vi "TCP.IP Server for Ripple Detection - Experiment 3.vi"() -> ()   [LabVIEW 2021]
doc: "Demonstrates how to set up a basic TCP connection, send data to the specified port once a connection has been established, and terminate the connection once the data has been sent. This VI is designed to stop if the TCP connection is terminated. The data sent in this example is an array of random numbers."
panel:
  in  "Number of row to read \nat a time":i32=10000
  in  "File Path":path
  out "Iteration terminal":i32
  in  "Stop 2":bool
  in  "Client Closed":string="The client VI closed the connection."
  in  "Stop":bool
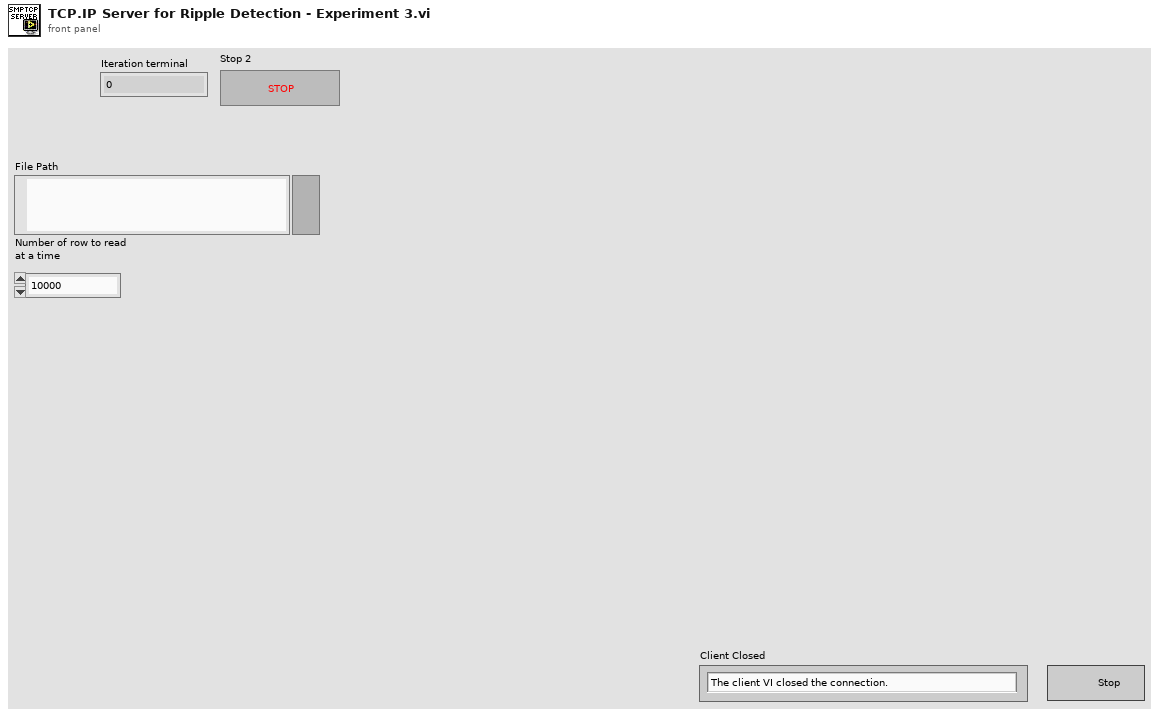
[diagram p1: front panel]
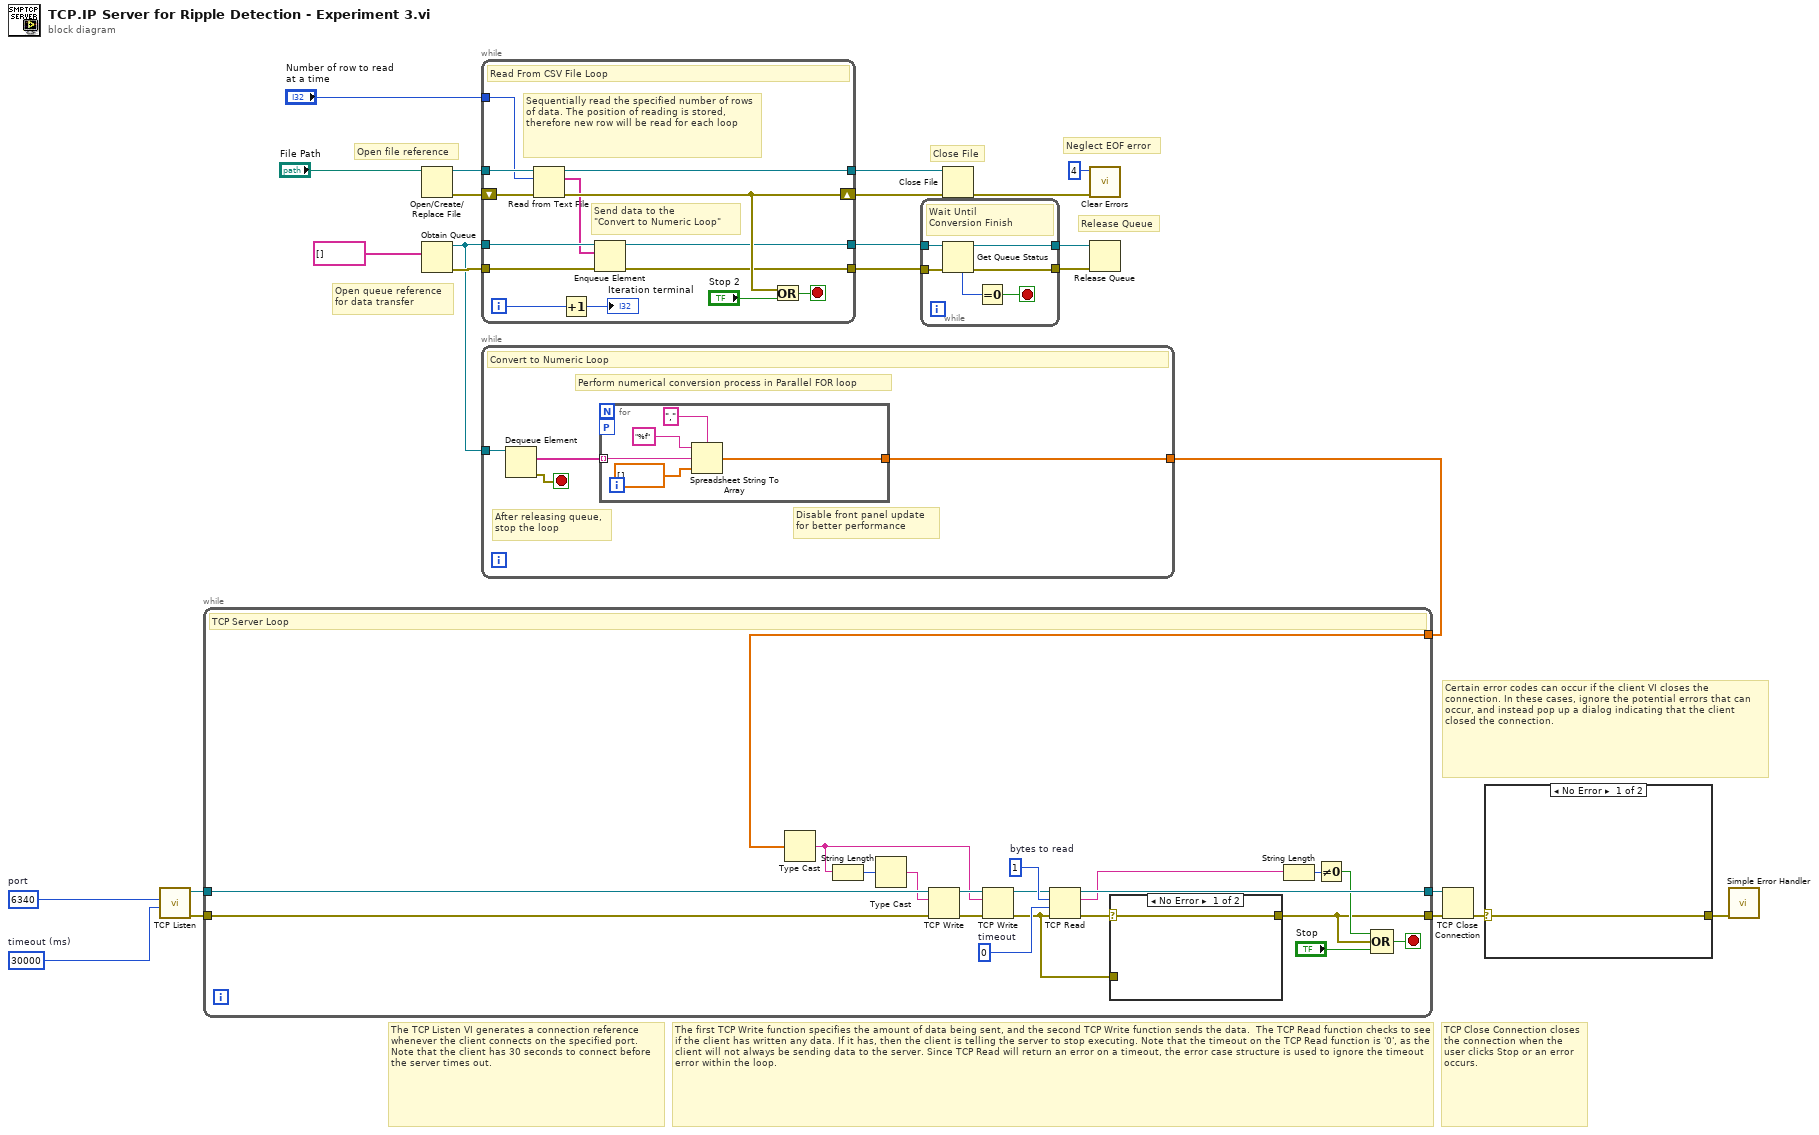
[diagram p0: block diagram]
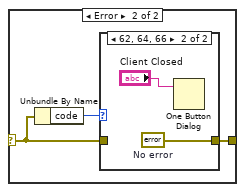
[diagram p2: hidden frame]
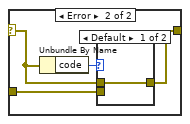
[diagram p4: hidden frame]
diagram:
  w17 = u16 6340  # port
  w18 = 30000  # timeout (ms)
  # "Neglect EOF error"
  # "Release Queue"
  # "Close File"
  # "Open queue reference\nfor data transfer"
  # "Open file reference"
  # "TCP Close Connection closes the connection when the user clicks Stop or an error occurs."
  # "The TCP Listen VI generates a connection reference whenever the client connects on the specified port. Note that the client has 30 seconds to connect before the server times out."
  # "Certain error codes can occur if the client VI closes the connection. In these cases, ignore the potential errors that can occur, and instead pop up a dialog indicating that the client closed the connection."
  # "The first TCP Write function specifies the amount of data being sent, and the second TCP Write function sends the data.  The TCP Read function checks to see if the client has written any data. If it has, then the client is telling the server to stop executing. Note that the timeout on the TCP Read function is '0', as the client will not always be sending data to the server. Since TCP Read will return an error on a timeout, the error case structure is used to ignore the timeout error within the loop."
  n1 = call <vilib>:"TCP Listen.vi"("timeout ms (wait forever: -1)"=w18, "port"=w17) -> ("error out"=w19:errorcluster, "connection ID"=w20:refnum<k5>)  [unwired: 5 in, 3 out]
  n2 = Open/Create/Replace File(file path (use dialog)="File Path") -> (refnum out=w14:refnum<file>, error out=w13:errorcluster)  [unwired: 5 in, 1 out]
  n3 = Obtain Queue(element data type=string[] [] ("形式文字列")) -> (queue out=w6:refnum<queue>, error out=w7:errorcluster)  [unwired: 4 in, 1 out]
  n4 = while {
    tunnel: w14 -> [w38]
    tunnel: [w36] -> w11
    shift-right: [w31] -> w10
    shift-left: w13 -> [w37]
    tunnel: "Number of row to read \nat a time" -> [w32]
    tunnel: w6 -> [w30]
    tunnel: w7 -> [w29]
    tunnel: [w27] -> w5
    tunnel: [w26] -> w4
    i -> [w34]
    stop <- w35 stop-if-true
    # "Send data to the \n\"Convert to Numeric Loop\""
    # "Sequentially read the specified number of rows of data. The position of reading is stored, therefore new row will be read for each loop"
    # "Read From CSV File Loop"
    n5 = Read from Text File(file (use dialog)=w38, count=w32, error in=w37) -> (refnum out=w36:refnum<file>, text=w28:string[], error out=w31:errorcluster)  [unwired: 1 in, 1 out]
    n6 = Increment(x=w34) -> (x+1=→"Iteration terminal":i32)
    n7 = Enqueue Element(queue=w30, element=w28, error in (no error)=w29) -> (queue out=w27:refnum<queue>, error out=w26:errorcluster)  [unwired: 1 in, 1 out]
    n8 = Or(x=w31, y="Stop 2") -> (x .or. y?=w35:bool)
  }
  n9 = while {
    tunnel: w6 -> [w42]
    tunnel: [w39] -> w1
    stop <- w40 stop-if-true
    # "Disable front panel update \nfor better performance"
    # "After releasing queue,\nstop the loop"
    # "Perform numerical conversion process in Parallel FOR loop"
    # "Convert to Numeric Loop"
    n10 = Dequeue Element(queue=w42) -> (element=w41:string[], error out=w40:errorcluster)  [unwired: 2 in, 2 out]
    n11 = for "Forループ" {
      tunnel: w41 -> [w45] mode=indexing
      tunnel: [w43] -> w39
      workers-P: _ -> [_]
      n12 = Spreadsheet String To Array(delimiter (Tab)="," ("デリミタ（タブ）"), format string="%f" ("形式文字列"), spreadsheet string=w45, array type (2D Dbl)=dbl[] []) -> (array=w43:dbl[])
    }
  }
  n13 = while {
    tunnel: [w50] -> w23
    tunnel: [w56] -> w24
    tunnel: w20 -> [w67]
    tunnel: w19 -> [w60]
    tunnel: w1 -> [w48]
    stop <- w61 stop-if-true
    w55 = 0  # timeout
    w58 = 1  # bytes to read
    # "TCP Server Loop"
    n14 = Type Cast(x=w48) -> (*(type *) &x=w62:string)  [unwired: 1 out]
    n15 = String Length(string=w62) -> (length=w64:i32)
    n16 = Type Cast(x=w64) -> (*(type *) &x=w63:string)  [unwired: 1 out]
    n17 = TCP Write(connection ID=w67, data in=w63, error in (no error)=w60) -> (connection ID out=w66:refnum<k5>, error out=w65:errorcluster)  [unwired: 2 out]
    n18 = TCP Write(connection ID=w66, data in=w62, error in (no error)=w65) -> (connection ID out=w57:refnum<k5>, error out=w49:errorcluster)  [unwired: 2 out]
    n19 = TCP Read(connection ID=w57, bytes to read=w58, error in (no error)=w49, 9:w55) -> (connection ID out=w56:refnum<k5>, data out=w53:string, error out=w51:errorcluster)  [unwired: 1 out]
    n20 = case shown="No Error" w51 {
      selector: w51 -> [w68 w71]
      tunnel: [w68 w69] -> w50
      tunnel: w49 -> [_ w70]
      frame No Error {
      }
      frame Error {
        n21 = Unbundle By Name(w71) -> ("code"=w72:i32)
        n22 = case shown="Default" w72 {
          tunnel: w71 -> [w73 _]
          tunnel: w70 -> [_ w74]
          tunnel: [w73 w74] -> w69
          frame Default {
          }
          frame 56 {
          }
        }
      }
    }
    n23 = String Length(string=w53) -> (length=w54:i32)
    n24 = Not Equal To 0?(x=w54) -> (x != 0?=w52:bool)
    n25 = Compound Arithmetic op=OR(w52, w50, "Stop") -> (w61:bool)
  }
  n26 = while {
    tunnel: w5 -> [w80]
    tunnel: w4 -> [w79]
    tunnel: [w76] -> w2
    tunnel: [w75] -> w3
    stop <- w77 stop-if-true
    # "Wait Until \nConversion Finish"
    n27 = Get Queue Status(queue=w80, error in (no error)=w79) -> (queue out=w76:refnum<queue>, error out=w75:errorcluster, # elements in queue=w78:i32)  [unwired: 1 in, 5 out]
    n28 = Equal To 0?(x=w78) -> (x = 0?=w77:bool)
  }
  n29 = Close File(refnum=w11, error in=w10) -> (error out=w9:errorcluster)  [unwired: 1 out]
  n30 = call <vilib>:"Clear Errors.vi"("error in (no error)"=w9, "specific error code to clear (0: all)"=4) -> ()  [unwired: 4 in, 2 out]
  n31 = Release Queue(queue=w2, error in (no error)=w3) -> ()  [unwired: 1 in, 3 out]
  n32 = TCP Close Connection(connection ID=w24, error in (no error)=w23) -> (error out=w22:errorcluster)  [unwired: 2 out]
  n33 = case shown="No Error" w22 {
    selector: w22 -> [w81 w83]
    tunnel: [w81 w82] -> w21
    frame No Error {
    }
    frame Error {
      n34 = Unbundle By Name(w83) -> ("code"=w84:i32)
      n35 = case shown="62, 64, 66" w84 {
        tunnel: w83 -> [w85 _]
        tunnel: [w85 w87] -> w82
        frame Default {
        }
        frame 62, 64, 66 {
          w87 = errorcluster {"status"=FALSE, "code"=0, "source"=""}  # No error
          n36 = One Button Dialog(message="Client Closed") -> ()  [unwired: 1 in, 1 out]
        }
      }
    }
  }
  n37 = call <vilib>:"Simple Error Handler.vi"("error in (no error)"=w21) -> ()  [unwired: 1 in, 8 out]
